vi "Logout.vi"(8 "error in (no error)":errorcluster, 10 "Authentication Inputs":T2, 11 "FormAuthentication in":refnum<class "FormAuthentication.lvclass">) -> (0 "error out":errorcluster, 2 "Authentication Outputs":T1, 3 "FormAuthentication out":refnum<class "FormAuthentication.lvclass">)   [LabVIEW 2020, in "HTTP Server.lvlib" / "FormAuthentication.lvclass"]
uses:
  FormAuthentication.lvclass
  Authentication Inputs.ctl
  Session/Session.lvclass
  <vilib>/IlluminatedG/IG HTTP Utils/HTTP Utils/Request/Request.lvclass
  User Provider/User Provider.lvclass
  Password Encoder/Password Encoder.lvclass
  Authentication Outputs.ctl
  User/User.lvclass
  FormAuthentication.lvclass/FormAuthentication.ctl
  HTTP Server.lvlib
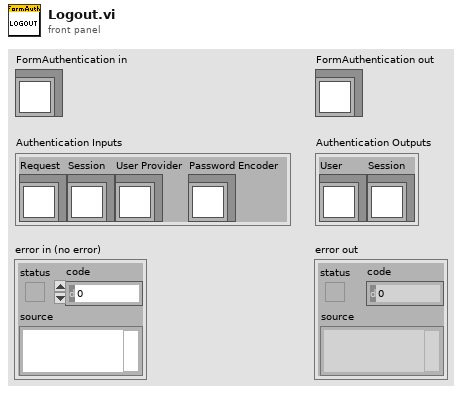
[diagram p1: front panel]
types:
  T1 = typedef "HTTP Server.lvlib/Authentication Outputs.ctl" = cluster{"User":refnum<class "User.lvclass">, "Session":refnum<class "Session.lvclass">}
  T2 = typedef "HTTP Server.lvlib/Authentication Inputs.ctl" = cluster{"Request":refnum<class "Request.lvclass">, "Session":refnum<class "Session.lvclass">, "User Provider":refnum<class "User Provider.lvclass">, "Password Encoder":refnum<class "Password Encoder.lvclass">}
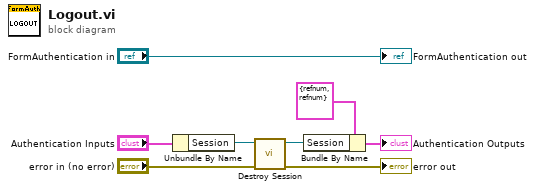
[diagram p0: block diagram]
diagram:
  n1 = Unbundle By Name("Authentication Inputs") -> ("Session"=w7:refnum<class "Session.lvclass">)
  n2 = call "Destroy Session.vi"("error in (no error)"="error in (no error)", "Session in"=w7) -> ("error out"=→"error out":errorcluster, "Session out"=w2:refnum<class "Session.lvclass">)  [unwired: 8 in]
  n3 = Bundle By Name(cluster=T1 {"User"=refnum, "Session"=refnum} ("Authentication Outputs"), "Session"=w2) -> (→"Authentication Outputs":T1)
  "FormAuthentication out" <- "FormAuthentication in"
